vi "AdafruitSeesawEncoder.vi"() -> ()   [LabVIEW 2020, in "CTI-Scratchpad.lvlib"]
uses:
  CTI-Scratchpad.lvlib
  CTI/Identity.ctl
  CTI/Error Reporting.ctl
  CTI/I2C Address.ctl
  CTI/GPIO Number.ctl
  CTI/I2C Number.ctl
  CTI/Session/Session.lvclass
  CTI/VisaComms/VisaComms.lvclass
  CTI/CTI.lvlib
  CTI-Peripheral/AdaFruit-Seesaw/AdaFruit-Seesaw.lvclass
panel:
  in  "Brightness":u8=20
  out "error out 2":errorcluster
  out "Button Pressed":bool
  out "GPIO":u32 format="%.0x"
  in  "Color Box":u32(colorbox)=6618880
  out "Encoder":i32
  in  "Stop":bool
  out "loop":i32
  out "Identity":T1
  in  "Grove Connector":enum16{"I2C0", "I2C1"}(ring)
  out "error out":errorcluster
  in  "Port":refnum<visa-resource-name>="COM4"
  # "https://labviewcommunitytraining.github.io/www/en/course_simple_grove_examples/v1.0/gadgets-nav.html#neopixel-ring"
  # "https://www.adafruit.com/product/5880"
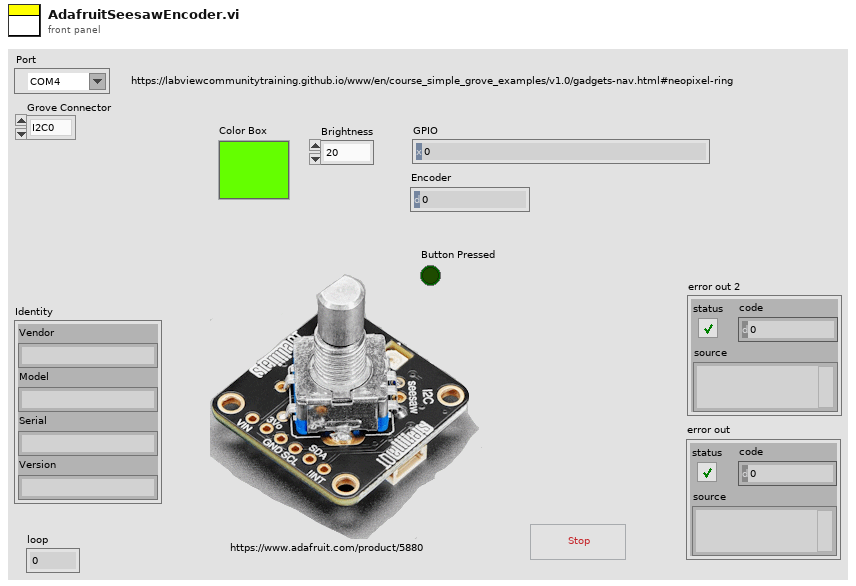
[diagram p1: front panel]
types:
  T1 = typedef "CTI.lvlib/Identity.ctl" = cluster{"Vendor":string, "Model":string, "Serial":string, "Version":string}
  T2 = typedef "CTI.lvlib/I2C Address.ctl" = u8
  T3 = typedef "CTI.lvlib/Error Reporting.ctl" = enum16{"Minimal", "Moderate", "Full"}
  T4 = typedef "CTI.lvlib/I2C Number.ctl" = i8
  T5 = typedef "CTI.lvlib/GPIO Number.ctl" = i8
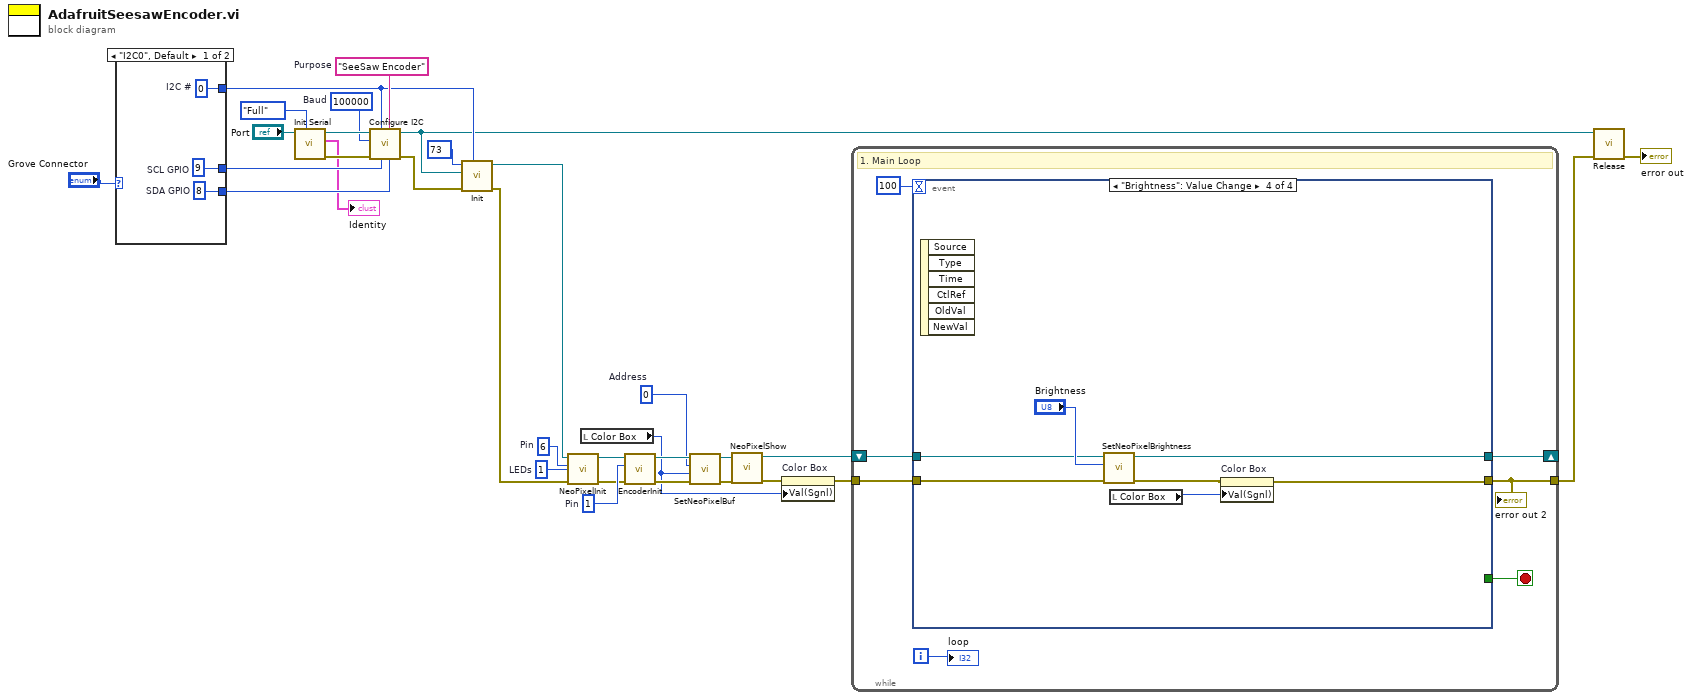
[diagram p0: block diagram]
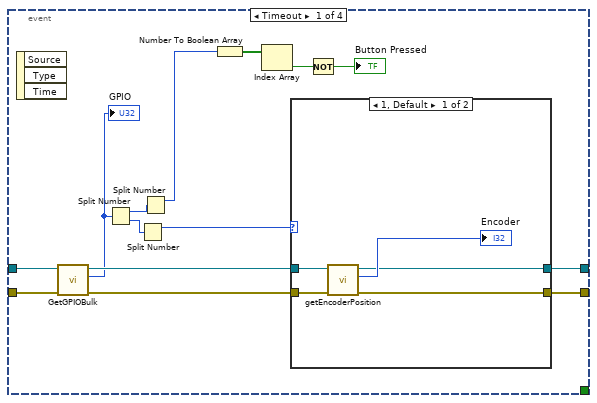
[diagram p2: hidden frame]
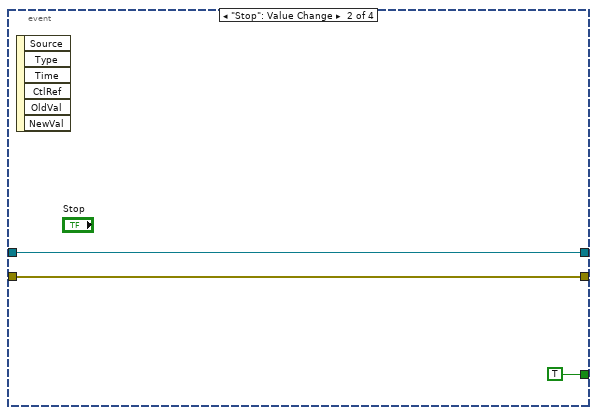
[diagram p4: hidden frame]
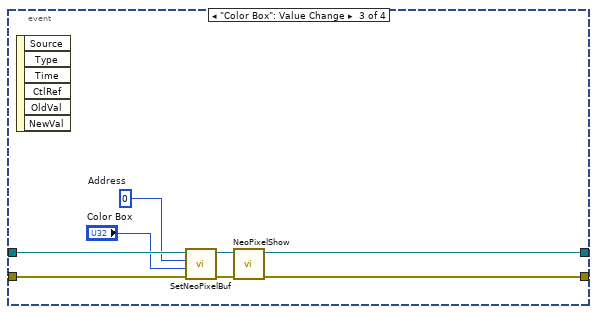
[diagram p5: hidden frame]
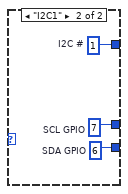
[diagram p6: hidden frame]
diagram:
  w1 = u8 1  # LEDs
  w9 = u16 0  # Address
  w13 = u8 1  # Pin
  w15 = u8 6  # Pin
  w27 = "SeeSaw Encoder"  # Purpose
  w28 = u32 100000  # Baud
  n1 = case shown="\"I2C0\", Default" "Grove Connector" {
    tunnel: [w35 w38] -> w25
    tunnel: [w34 w37] -> w24
    tunnel: [w33 w36] -> w20
    frame "I2C0", Default {
      w33 = T4 0  # I2C #
      w34 = T5 8  # SDA GPIO
      w35 = T5 9  # SCL GPIO
    }
    frame "I2C1" {
      w36 = T4 1  # I2C #
      w37 = T5 6  # SDA GPIO
      w38 = T5 7  # SCL GPIO
    }
  }
  n2 = call "Init Serial.vi"("Error Checking (Full)"=Error_Reporting."Full", "VISA resource name in"="Port") -> ("error out"=w29:errorcluster, "Identity"=→"Identity":T1, "Session"=w30:refnum<class "Session.lvclass">)  [unwired: 7 in]
  n3 = call "Configure I2C.vi"("SDA GPIO"=w24, "Purpose (\"I2C\")"=w27, "SCL GPIO"=w25, "I2C #"=w20, "error in (no error)"=w29, "Baud"=w28, "Session in"=w30) -> ("error out"=w18:errorcluster, "Session out"=w19:refnum<class "Session.lvclass">)  [unwired: 3 in]
  n4 = call "Init.vi"("I2C #"=w20, "error in (no error)"=w18, "Session In"=w19, "Address"=T2 73) -> ("error out"=w16:errorcluster, "AdaFruit-Seesaw out"=w17:refnum<class "AdaFruit-Seesaw.lvclass">)  [unwired: 6 in]
  n5 = call "NeoPixelInit.vi"("error in (no error)"=w16, "LEDs"=w1, "Pin"=w15, "AdaFruit-Seesaw in"=w17) -> ("error out"=w12:errorcluster, "AdaFruit-Seesaw out"=w14:refnum<class "AdaFruit-Seesaw.lvclass">)  [unwired: 6 in]
  n6 = local read "Color Box"() -> (w3:u32)
  n7 = call "EncoderInit.vi"("error in (no error)"=w12, "Pin"=w13, "AdaFruit-Seesaw in"=w14) -> ("error out"=w10:errorcluster, "AdaFruit-Seesaw out"=w11:refnum<class "AdaFruit-Seesaw.lvclass">)  [unwired: 7 in]
  n8 = call "SetNeoPixelBuf.vi"("error in (no error)"=w10, "Color Box"=w3, "Address"=w9, "AdaFruit-Seesaw in"=w11) -> ("error out"=w8:errorcluster, "AdaFruit-Seesaw out"=w7:refnum<class "AdaFruit-Seesaw.lvclass">)  [unwired: 6 in]
  n9 = call "NeoPixelShow.vi"("error in (no error)"=w8, "AdaFruit-Seesaw in"=w7) -> ("error out"=w5:errorcluster, "AdaFruit-Seesaw out"=w6:refnum<class "AdaFruit-Seesaw.lvclass">)  [unwired: 8 in]
  n10 = property on="Color Box" class="ColBox"(error in=w5, "Val(Sgnl)"=w3) -> (error out=w4:errorcluster)  [unwired: 1 in, 1 out]
  n11 = while {
    tunnel: w4 -> [w44]
    tunnel: [w42] -> w22
    shift-right: [w39] -> _
    shift-left: w6 -> [w45]
    i -> [w43]
    stop <- w40 stop-if-true
    # "1. Main Loop"
    n12 = event shown="[3] \"Brightness\": Value Change" {
      selector: _ -> [_ _ _ _]
      dyn-events: _ -> [_ _ _ _]
      timeout: 100 -> [_ _ _ _]
      tunnel: w45 -> [w57 w67 w74 w83]
      tunnel: w44 -> [w58 w68 w75 w82]
      tunnel: [w59 w68 w73 w80] -> w42
      tunnel: [_ TRUE _ _] -> w40
      tunnel: [w46 w67 w70 w79] -> w39
      event Timeout {
        n13 = event-data() -> ()  [unwired: 1 in, 3 out]
        n14 = call "GetGPIOBulk.vi"("error in (no error)"=w58, "AdaFruit-Seesaw in"=w57) -> ("error out"=w55:errorcluster, "GPIO"=w53:u32, "AdaFruit-Seesaw out"=w56:refnum<class "AdaFruit-Seesaw.lvclass">)  [unwired: 7 in]
        "GPIO" <- w53
        n15 = Split Number(x=w53) -> (hi(x)=w50:u16, lo(x)=w54:u16)
        n16 = Split Number(x=w54) -> (hi(x)=w52:u8)  [unwired: 1 out]
        n17 = Split Number(x=w50) -> (hi(x)=w51:u8)  [unwired: 1 out]
        n18 = Number To Boolean Array(number=w51) -> (Boolean array=w49:bool[])
        n19 = Index Array(array=w49) -> (element=w48:bool)  [unwired: 1 in]
        n20 = case shown="1, Default" w52 {
          tunnel: [w64 w66] -> w59
          tunnel: w56 -> [w62 w65]
          tunnel: w55 -> [w61 w66]
          tunnel: [w60 w65] -> w46
          frame 1, Default {
            n21 = call "getEncoderPosition.vi"("error in (no error)"=w61, "AdaFruit-Seesaw in"=w62) -> ("error out"=w64:errorcluster, "Position"=→"Encoder":i32, "AdaFruit-Seesaw out"=w60:refnum<class "AdaFruit-Seesaw.lvclass">)  [unwired: 7 in]
          }
          frame 0, 197 {
            # "Not changed"
          }
        }
        n22 = Not(x=w48) -> (.not. x?=→"Button Pressed":bool)
      }
      event "Stop": Value Change {
        n23 = event-data() -> ()  [unwired: 1 in, 6 out]
      }
      event "Color Box": Value Change {
        w71 = u16 0  # Address
        n24 = event-data() -> ()  [unwired: 1 in, 6 out]
        n25 = call "SetNeoPixelBuf.vi"("error in (no error)"=w75, "Color Box"="Color Box", "Address"=w71, "AdaFruit-Seesaw in"=w74) -> ("error out"=w76:errorcluster, "AdaFruit-Seesaw out"=w77:refnum<class "AdaFruit-Seesaw.lvclass">)  [unwired: 6 in]
        n26 = call "NeoPixelShow.vi"("error in (no error)"=w76, "AdaFruit-Seesaw in"=w77) -> ("error out"=w73:errorcluster, "AdaFruit-Seesaw out"=w70:refnum<class "AdaFruit-Seesaw.lvclass">)  [unwired: 8 in]
      }
      event "Brightness": Value Change {
        n27 = event-data() -> ()  [unwired: 1 in, 6 out]
        n28 = call "SetNeoPixelBrightness.vi"("error in (no error)"=w82, "Brightness"="Brightness", "AdaFruit-Seesaw in"=w83) -> ("error out"=w81:errorcluster, "AdaFruit-Seesaw out"=w79:refnum<class "AdaFruit-Seesaw.lvclass">)  [unwired: 7 in]
        n29 = local read "Color Box"() -> (w78:u32)
        n30 = property on="Color Box" class="ColBox"(error in=w81, "Val(Sgnl)"=w78) -> (error out=w80:errorcluster)  [unwired: 1 in, 1 out]
      }
    }
    "error out 2" <- w42
    "loop" <- w43
  }
  n31 = call-dynamic "Release.vi"("error in (no error)"=w22, "Session in"=w19) -> ("error out"=→"error out":errorcluster)  [unwired: 9 in]
